vi "사인파형생성.vi"() -> (0 "경로":path, 1 "웨이브폼 그래프":dbl[](graph))   [LabVIEW 2014]
uses:
  <vilib>/Utility/file.llb/Write To Spreadsheet File (DBL).vi
  <vilib>/Analysis/NI_AALBase.lvlib
panel:
  in  "취소 버튼":bool
  in  "확인 버튼":bool
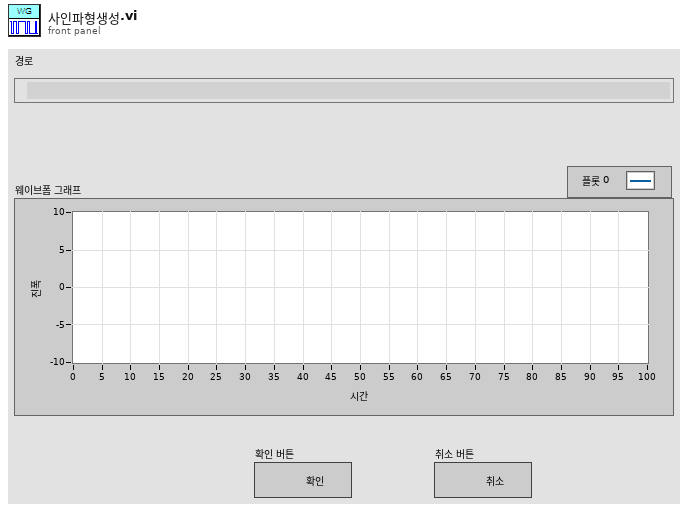
[diagram p1: front panel]
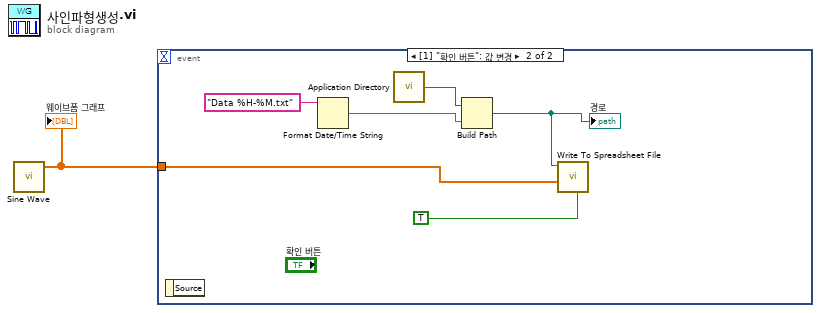
[diagram p0: block diagram]
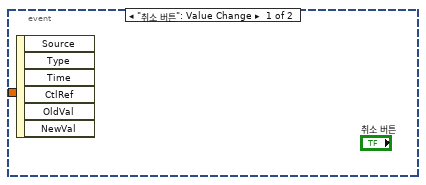
[diagram p2: hidden frame]
diagram:
  n1 = call <vilib>:"Sine Wave.vi"() -> ("sine wave"=w1:dbl[])  [unwired: 5 in, 2 out]
  "웨이브폼 그래프" <- w1
  n2 = event shown="[1] \"확인 버튼\": 값 변경" {
    selector: _ -> [_ _]
    dyn-events: _ -> [_ _]
    timeout: _ -> [_ _]
    tunnel: w1 -> [_ w7]
    event "취소 버튼": Value Change {
      n3 = event-data() -> ()  [unwired: 1 in, 6 out]
    }
    event "확인 버튼": Value Change {
      n4 = event-data() -> ()  [unwired: 1 in, 1 out]
      n5 = Format Date/Time String(time format string (%c)="Data %H-%M.txt" ("시간 포맷 문자열 (%c)")) -> (date/time string=w4:string)  [unwired: 2 in]
      n6 = call <vilib>:"Application Directory.vi"() -> ("Application Directory"=w3:path)
      n7 = Build Path(base path=w3, name or relative path=w4) -> (appended path=w2:path)
      "경로" <- w2
      n8 = call-poly <vilib>:"Write To Spreadsheet File.vi"("transpose? (no:F)"=TRUE, "1D data"=w7, "file path (dialog if empty)"=w2) -> ()  [unwired: 5 in, 1 out]
    }
  }
